vi "dbc-get-signal-value.vi"(7 "frame.tag":string, 8 "error in (no error)":errorcluster, 9 "bit.len":i32, 10 "start.pos":i32, 11 "dbc in":refnum<class "dbc.lvclass">) -> (0 "error out":errorcluster, 2 "Numeric":u32, 3 "dbc out":refnum<class "dbc.lvclass">)   [LabVIEW 2015]
uses:
  class.can.table/CANtable.lvclass
  dbc.lvclass
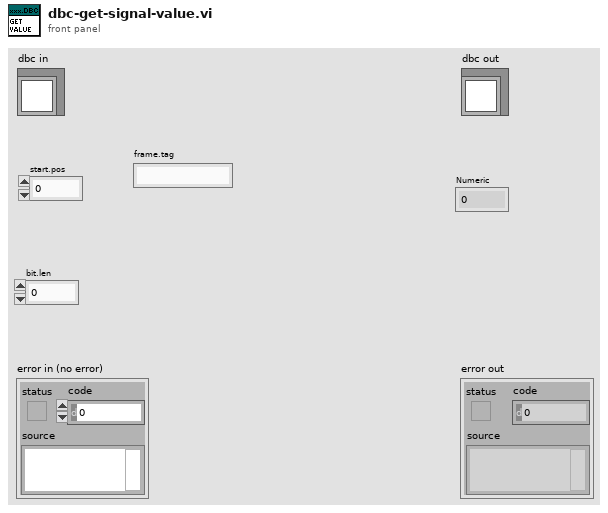
[diagram p1: front panel]
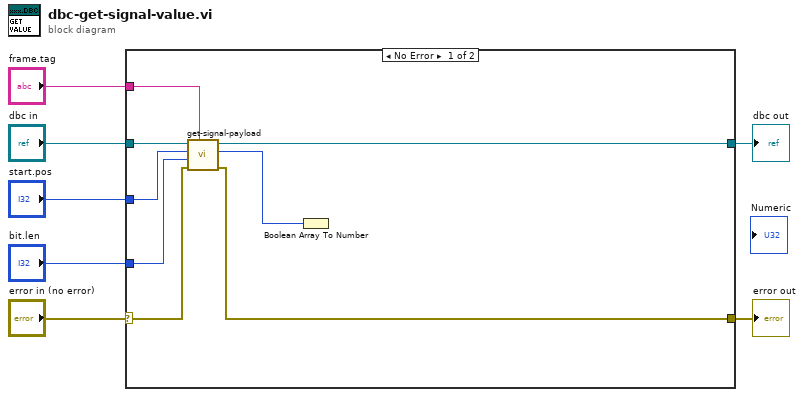
[diagram p0: block diagram]
diagram:
  n1 = case shown="No Error" "error in (no error)" {
    selector: "error in (no error)" -> [w10 w17]
    tunnel: [w9 w17] -> w6
    tunnel: [w14 w16] -> w4
    tunnel: "dbc in" -> [w15 w16]
    tunnel: "frame.tag" -> [w13 _]
    tunnel: "start.pos" -> [w12 _]
    tunnel: "bit.len" -> [w11 _]
    frame No Error {
      n2 = call "get-signal-payload.vi"("tag"=w13, "error in (no error)"=w10, "bit.len"=w11, "start.pos"=w12, "CANtable in"=w15) -> ("error out"=w9:errorcluster, "payload"=w8:u32, "CANtable out"=w14:refnum<class "dbc.lvclass">)  [unwired: 4 in]
      n3 = Boolean Array To Number(Boolean array=w8) -> ()  [unwired: 1 out]
    }
    frame Error {
    }
  }
  "error out" <- w6
  "dbc out" <- w4
